vi "ShowAnalysisData.vi"(8 "error in (no error)":errorcluster, 10 "Analysis in":refnum<class "Analysis.lvclass">, 11 "Table Control":refnum<vi>) -> (0 "error out":errorcluster)   [LabVIEW 2017]
doc: "Loads the Analysis Data from the AnalysisObject and displays the data in the Table"
uses:
  MSControl/Classes/Analysis/Analysis.lvclass
  <vilib>/Utility/miscctls.llb/LVRowAndColumnUnsignedTypeDef.ctl
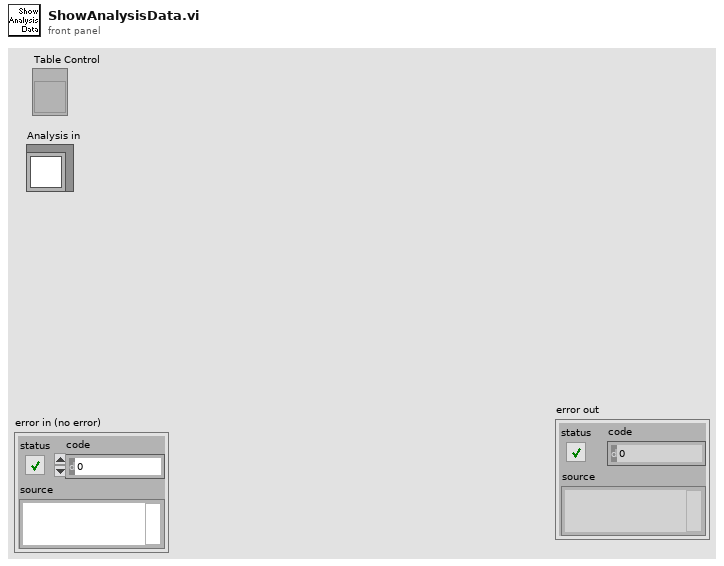
[diagram p1: front panel]
types:
  T1 = typedef "LVRowAndColumnUnsignedTypeDef.ctl" = cluster{"Row":u32, "Column":u32}
  T2 = typedef "AnalysisDataArray.ctl" = cluster{"analysis data":string[][]}[]
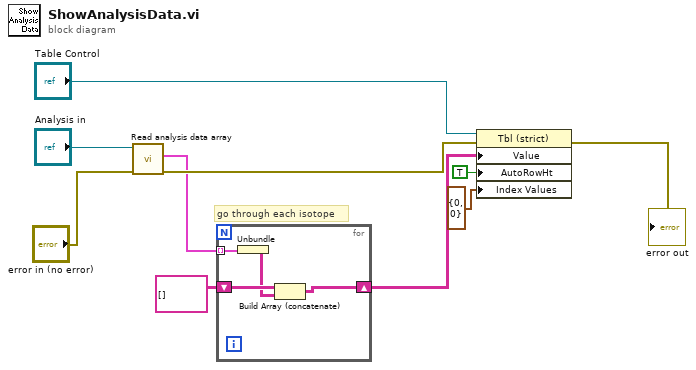
[diagram p0: block diagram]
diagram:
  # "go through each isotope"
  n1 = call-dynamic "Read analysis data array.vi"("error in (no error)"="error in (no error)", "Analysis in"="Analysis in") -> ("error out"=w6:errorcluster, "analysis data array"=w4:T2)  [unwired: 7 in, 1 out]
  n2 = for {
    tunnel: w4 -> [w12] mode=indexing
    shift-right: [w13] -> w2
    shift-left: string[][] [] -> [w14]
    n3 = Unbundle(w12) -> ("analysis data"=w11:string[][])
    n4 = Build Array (concatenate)(w14, w11) -> (w13:string[][])
  }
  n5 = property class="Tbl (strict)"(reference="Table Control", error in=w6, "Value"=w2, "AutoRowHt"=TRUE ("Autosizing Row Height"), "Index Values"=T1 {"Row"=0, "Column"=0}) -> (error out=→"error out":errorcluster)  [unwired: 1 out]
